vi "setUp.vi"(8 "error in":errorcluster, 11 "reference in":refnum<class "Embedded Data Logger Windows System Tests.lvclass">) -> (0 "error out":errorcluster, 3 "reference out":refnum<class "Embedded Data Logger Windows System Tests.lvclass">)   [LabVIEW 2027, in "Embedded Data Logger Windows System Tests.lvclass"]
doc: "setUp runs prior to the test method during test execution. Use this method to initialize any object data required by your tests."
uses:
  Embedded Data Logger Windows System Tests.lvclass
  C:/Program Files/National Instruments/LabVIEW 2027/vi.lib/addons/_JKI Toolkits/VI Tester/TestCase.llb/TestCase.lvclass
  <vilib>/addons/_JKI Toolkits/VI Tester/TestCase.llb/TestCase.lvclass
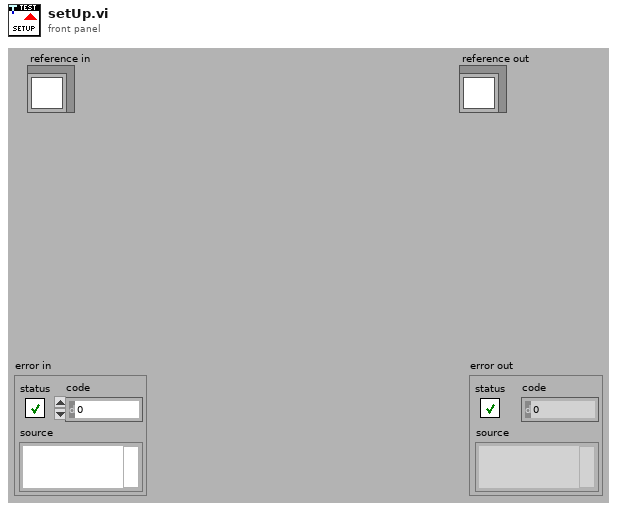
[diagram p1: front panel]
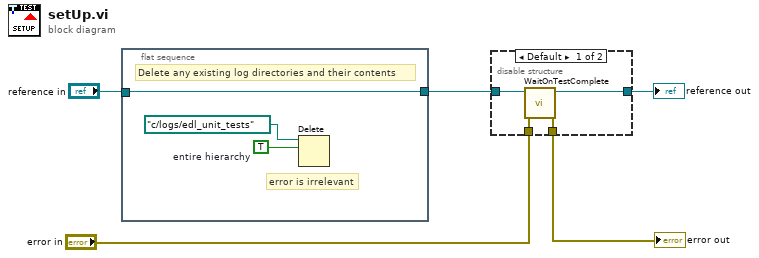
[diagram p0: block diagram]
diagram:
  n1 = flat-sequence {
    tunnel: [w8] -> w1
    tunnel: "reference in" -> [w8]
    frame #0 {
      w7 = TRUE  # entire hierarchy
      # "error is irrelevant"
      # "Delete any existing log directories and their contents"
      n2 = Delete(path (use dialog)=path "c:/logs/edl_unit_tests" ("file path"), entire hierarchy (F)=w7) -> ()  [unwired: 3 in, 3 out]
    }
  }
  n3 = disable-structure shown="Default" {
    disable-tunnel: "error in" -> [w12 w13]
    disable-tunnel: [w11 w13] -> w5
    disable-tunnel: [w10 w14] -> w4
    disable-tunnel: w1 -> [w9 w14]
    frame condition #0 (active) {
      n4 = call <vilib>:"WaitOnTestComplete.vi"("error in (no error)"=w12, "TestCase in"=w9) -> ("error out"=w11:errorcluster, "TestCase out"=w10:refnum<class "Embedded Data Logger Windows System Tests.lvclass">)  [unwired: 8 in]
    }
    frame condition #1 {
    }
  }
  "error out" <- w5
  "reference out" <- w4
